vi "ZDataVIS_grab_IV_itx.vi"(4 "offset":i32, 6 "decimate files (1 for no)":i32=1, 9 "pattern":string="*.itx", 11 "File or Folder Path":path=path "G:/My Drive/ansom/Data/PPMS2/SA03008L.20190612/030_phi_90_Vamp_bg=30_IV_Testing/SA03008L.20190612.000014.itx") -> (1 "\"notes \"":string[](array[string]), 2 "Index, Wavenames":string[][](table)=[["0", "'time.SA03008L.20190612.000014'\n"], ["1", "'temp.SA03008L.20190612.000014'\n"], ["2", "'B.SA03008L.20190612.000014'\n"], ["3", "'Brate.SA03008L.20190612.000014'\n"], ["4", "'Lockin1.SA03008L.20190612.000014'\n"], ["5", "'Lockin2.SA03008L.20190612.000014'\n"], ["6", "'Lockin3.SA03008L.20190612.000014'\n"], ["7", "'Lockin4.SA03008L.20190612.000014'\n"], ["8", "'Lockin5.SA03008L.20190612.000014'\n"], ["9", "'Lockin6.SA03008L.20190612.000014'\n"], ["10", "'AO1.SA03008L.20190612.000014'\n"], ["11", "'AO2.SA03008L.20190612.000014'\n"], ["12", "'AO3.SA03008L.20190612.000014'\n"], ["13", "'AO4.SA03008L.20190612.000014'\n"], ["14", "'AO5.SA03008L.20190612.000014'\n"], ["15", "'AO6.SA03008L.20190612.000014'\n"], ["16", "'AO7.SA03008L.20190612.000014'\n"], ["17", "'AO8.SA03008L.20190612.000014'\n"], ["", ""]], 3 "All ITX data..":dbl[][][](array[numeric]))   [LabVIEW 2016]
uses:
  <vilib>/addons/WireFlow/_WF_ProgressBar.llb/ProgressBar_WireFlow.lvclass
  <userlib>/LevyLab/LV to ITX/LVtoITX.lvclass
panel:
  out "total megabyte estimate":dbl
  out "size(s)":i32[](array[numeric])
  out "megabytes in output":dbl
  out "WF-ProgressBar out":refnum<class "ProgressBar_WireFlow.lvclass">
  in  "Generate Folder Index File?":bool
  in  "Use Folder Index File?":bool
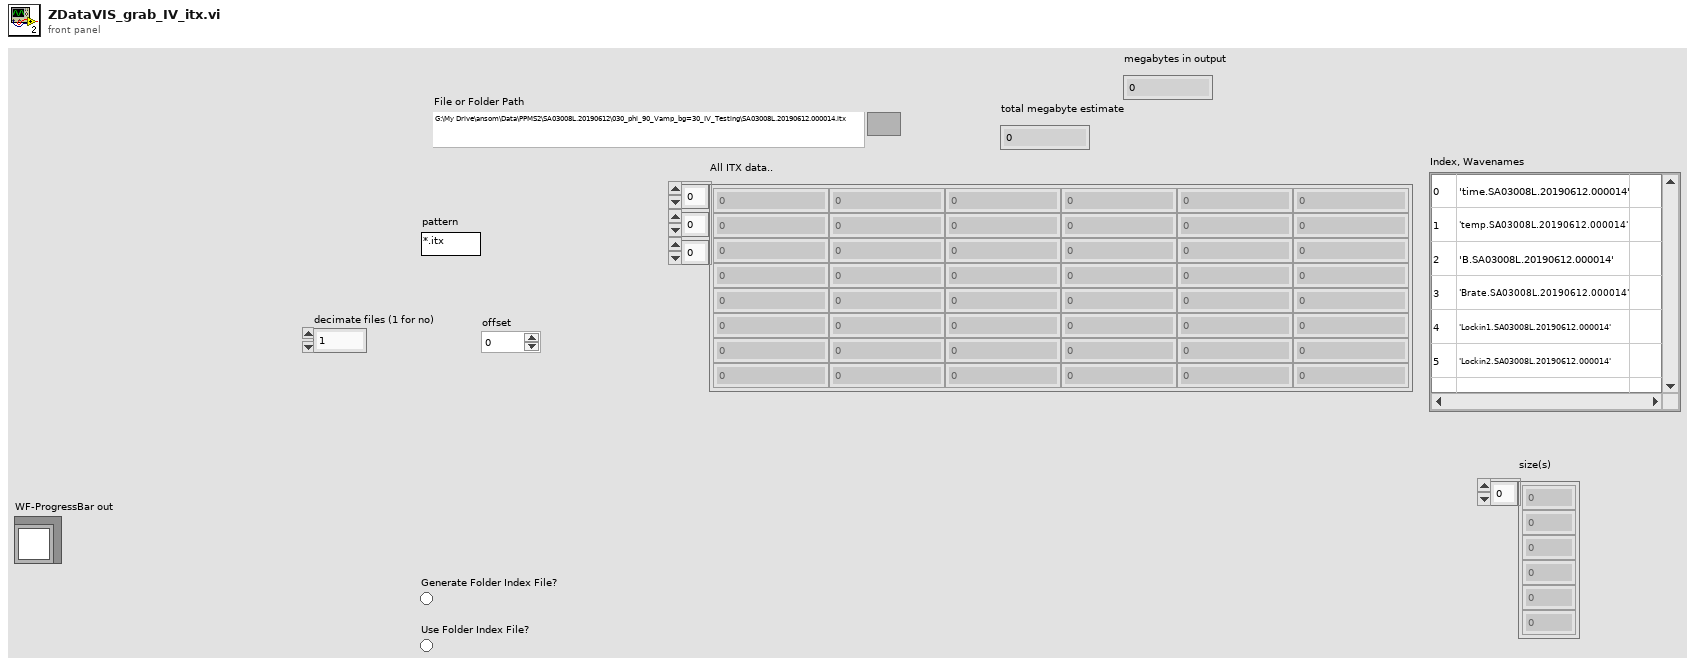
[diagram p1: front panel]
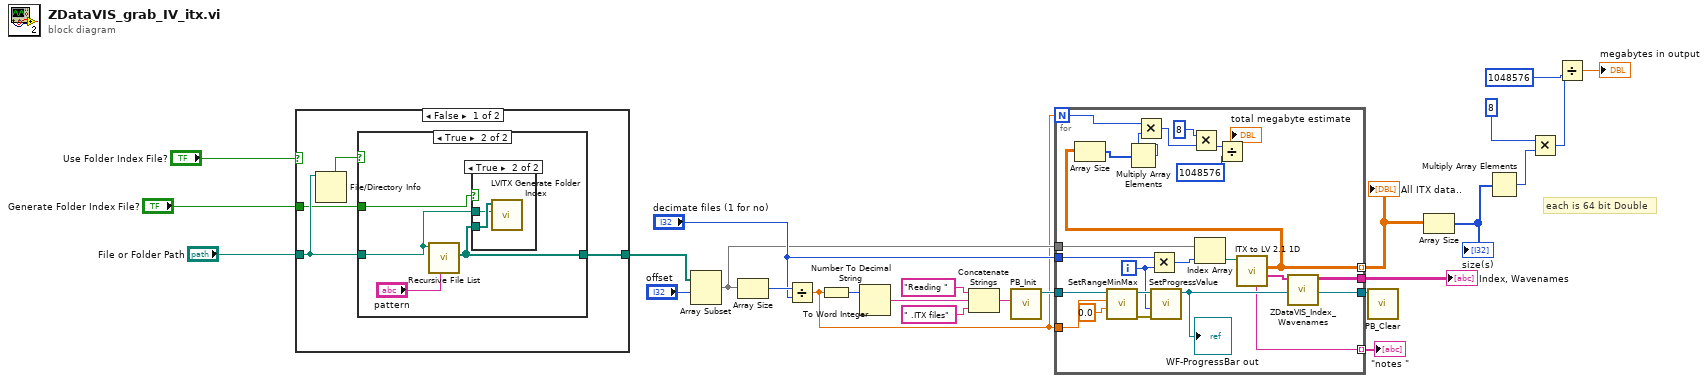
[diagram p0: block diagram]
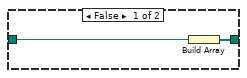
[diagram p2: hidden frame]
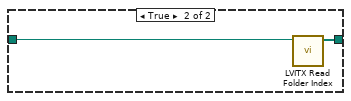
[diagram p4: hidden frame]
diagram:
  # "each is 64 bit Double"
  n1 = case shown="False" "Use Folder Index File?" {
    tunnel: [w27 w38] -> w20
    tunnel: "File or Folder Path" -> [w29 w39]
    tunnel: "Generate Folder Index File?" -> [w26 _]
    frame False {
      n2 = File/Directory Info(path=w29) -> (directory=w28:bool)  [unwired: 1 in, 6 out]
      n3 = case shown="True" w28 {
        tunnel: [w31 w34] -> w27
        tunnel: w29 -> [w30 w33]
        tunnel: w26 -> [_ w32]
        frame False {
          n4 = Build Array(w30) -> (w31:path[])
        }
        frame True {
          n5 = call <vilib>:"Recursive File List.vi"("pattern"="pattern", "Folder Path"=w33) -> ("All Files in Dir"=w34:path[])  [unwired: 5 in, 4 out]
          n6 = case shown="True" w32 {
            tunnel: w34 -> [_ w37]
            tunnel: w33 -> [_ w36]
            frame False {
            }
            frame True {
              n7 = call <userlib>:"LVITX Generate Folder Index.vi"("File or Folder Path"=w36, "All Files in Dir"=w37) -> ()  [unwired: 9 in, 1 out]
            }
          }
        }
      }
    }
    frame True {
      n8 = call <userlib>:"LVITX Read Folder Index.vi"("File or Folder Path"=w39) -> ("Files"=w38:path[])  [unwired: 9 in, 1 out]
    }
  }
  n9 = Array Subset(array=w20, index="offset") -> (w18:path[])  [unwired: 1 in]
  n10 = Array Size(array=w18) -> (size(s)=w21:i32)
  n11 = Divide(x=w21, y="decimate files (1 for no)") -> (x/y=w2:dbl)
  n12 = To Word Integer(number=w2) -> (16bit integer=w12:i16)
  n13 = Number To Decimal String(number=w12) -> (decimal integer string=w11:string)  [unwired: 1 in]
  n14 = Concatenate Strings("Reading " ("title (\"Progress\")"), w11, " .ITX files" ("title (\"Progress\")")) -> (w10:string)
  n15 = call <vilib>:"PB_Init.vi"("title (\"Progress\")"=w10) -> ("WF-ProgressBar out"=w15:refnum<class "ProgressBar_WireFlow.lvclass">)  [unwired: 9 in, 1 out]
  n16 = for {
    N: w2 -> [w47]
    tunnel: "decimate files (1 for no)" -> [w62]
    tunnel: w18 -> [w61]
    tunnel: [w49] -> w3 mode=indexing
    tunnel: [w57] -> w17
    tunnel: [w53] -> w16
    tunnel: w15 -> [w52]
    tunnel: w2 -> [w51]
    tunnel: [w40] -> w1 mode=indexing
    i -> [w50]
    n17 = call-dynamic "SetRangeMinMax.vi"("Min (0)"=0.0, "Max (1)"=w51, "WF-ProgressBar in"=w52) -> ("error out"=w55:errorcluster, "WF-ProgressBar out"=w54:refnum<class "ProgressBar_WireFlow.lvclass">)  [unwired: 7 in]
    n18 = Multiply(x=w62, y=w50) -> (x*y=w58:i32)
    n19 = call-dynamic "SetProgressValue.vi"("error in (no error)"=w55, "Value"=w50, "WF-ProgressBar in"=w54) -> ("WF-ProgressBar out"=w53:refnum<class "ProgressBar_WireFlow.lvclass">)  [unwired: 6 in, 2 out]
    "WF-ProgressBar out" <- w53
    n20 = Index Array(array=w61, index=w58) -> (element=w59:path)
    n21 = call <userlib>:"ITX to LV 2.1 1D.vi"("file (use dialog)"=w59) -> ("wave names"=w60:string[], "1D arrays"=w49:dbl[][], "Notes"=w40:string)  [unwired: 6 in, 2 out]
    n22 = Array Size(array=w49) -> (size(s)=w48:i32[])
    n23 = Multiply Array Elements(1:w48) -> (0:w46:i32)
    n24 = Multiply(x=w47, y=w46) -> (x*y=w45:i32)
    n25 = Multiply(x=8, y=w45) -> (x*y=w43:i32)
    n26 = Divide(x=w43, y=1048576) -> (x/y=→"total megabyte estimate":dbl)
    n27 = call "ZDataVIS_Index_Wavenames.vi"("wave names"=w60) -> ("Index, Wavenames"=w57:string[][])  [unwired: 10 in]
  }
  "All ITX data.." <- w3
  "Index, Wavenames" <- w17
  "\"notes \"" <- w1
  n28 = call-dynamic "PB_Clear.vi"("WF-ProgressBar in"=w16) -> ()  [unwired: 9 in, 2 out]
  n29 = Array Size(array=w3) -> (size(s)=w9:i32[])
  "size(s)" <- w9
  n30 = Multiply Array Elements(1:w9) -> (0:w7:i32)
  n31 = Multiply(x=8, y=w7) -> (x*y=w5:i32)
  n32 = Divide(x=w5, y=1048576) -> (x/y=→"megabytes in output":dbl)
